vi "Write XRay CArm.lvclass.vi"(8 "error in (no error)":errorcluster, 10 "XRay CArm.lvclass":refnum<class "XRay CArm.lvclass">, 11 "XRay Beam in":refnum<class "XRay Beam.lvclass">) -> (0 "error out":errorcluster, 3 "XRay Beam out":refnum<class "XRay Beam.lvclass">)   [LabVIEW 2026, in "XRay Beam.lvclass"]
uses:
  XRay Beam.lvclass
  XRay CArm/XRay CArm.lvclass
  XRay Beam.lvclass/XRay Beam.ctl
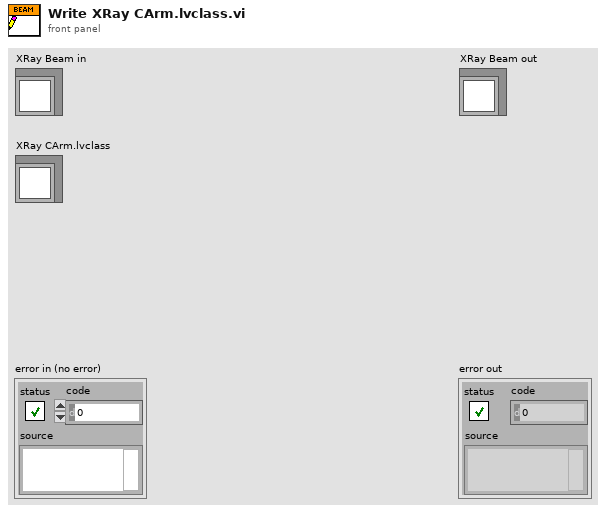
[diagram p1: front panel]
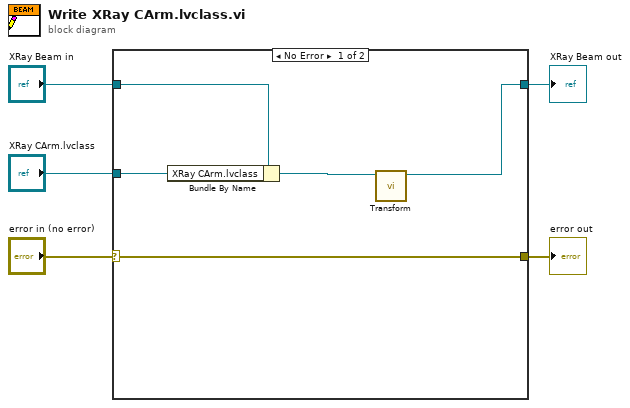
[diagram p0: block diagram]
diagram:
  n1 = case shown="No Error" "error in (no error)" {
    selector: "error in (no error)" -> [w10 w11]
    tunnel: [w10 w11] -> w4
    tunnel: [w6 w12] -> w2
    tunnel: "XRay Beam in" -> [w9 w12]
    tunnel: "XRay CArm.lvclass" -> [w8 _]
    frame No Error {
      n2 = Bundle By Name(cluster=w9, "XRay CArm.lvclass"=w8) -> (w7:refnum<class "XRay Beam.lvclass">)
      n3 = call-dynamic "Transform.vi"("XRay Beam in"=w7) -> ("XRay Beam out"=w6:refnum<class "XRay Beam.lvclass">)  [unwired: 9 in, 1 out]
    }
    frame Error {
    }
  }
  "error out" <- w4
  "XRay Beam out" <- w2
